vi "Get Element Info Variant.vi"(8 "error in (no error)":errorcluster, 11 "Data Type":variant) -> (0 "error out":errorcluster, 1 "Array Element Size":i32, 2 "Array Size":i32, 3 "Total Size":i32, 4 "Cluster Info":T1[](array[typedef]), 5 "Array":bool)   [LabVIEW 2021, in "CIF_NI_CIPC.lvlib"]
uses:
  CIF_NI_CIPC.lvlib
  <vilib>/CIF Foundation/CIF Utilities/DataTypes/Typedef/Cluster Info.ctl
  <vilib>/Utility/Data Type/Type Definitions/Data Type.ctl
  <vilib>/Utility/Data Type/NI_Data Type.lvlib
  <vilib>/CIF Foundation/CIF Utilities/DataTypes/DataTypes_CIF_U.lvlib
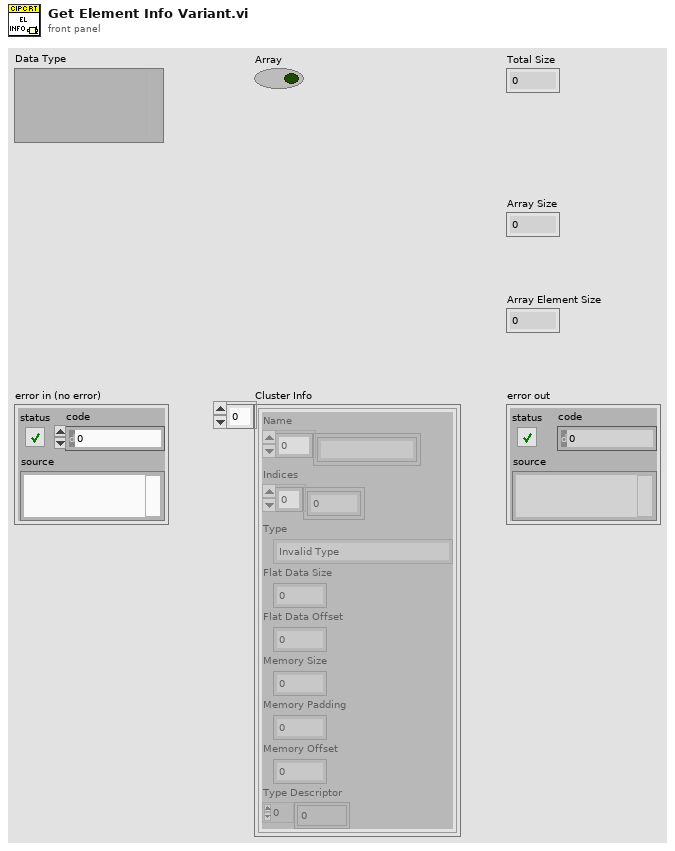
[diagram p1: front panel]
types:
  T1 = typedef "DataTypes_CIF_U.lvlib/Cluster Info.ctl" = cluster{"Name":string[], "Indices":i32[], "Type":T2, "Flat Data Size":u32, "Flat Data Offset":u32, "Memory Size":u32, "Memory Padding":u32, "Memory Offset":u32, "Type Descriptor":i16[]}
  T2 = typedef "NI_Data Type.lvlib/Data Type.ctl" = enum8{"Invalid Type", "Void", "I8", "I16", "I32", "I64", "U8", "U16", "U32", "U64", "Single Float", "Double Float", "Extended Float", "Single Complex", "Double Complex", "Extended Complex", "Enum U8", "Enum U16", "Enum U32", "Enum U64", "Single Float With Unit", "Double Float With Unit", "Extended Float With Unit", "Single Complex with Unit", "Double Complex with Unit", "Extended Complex with Unit", "Boolean", "String", "Path", "Picture", "Tag", "Array", "Cluster", "Variant", "LV Variant", "Waveform", "Timestamp", "Digital Waveform", "Digital Data", "ExpressData", "Refnum", "External Data", "VI", "Poly VI", "LabVIEW Class Instance", "Fixed Point", "Set Collection", "Map Collection"}
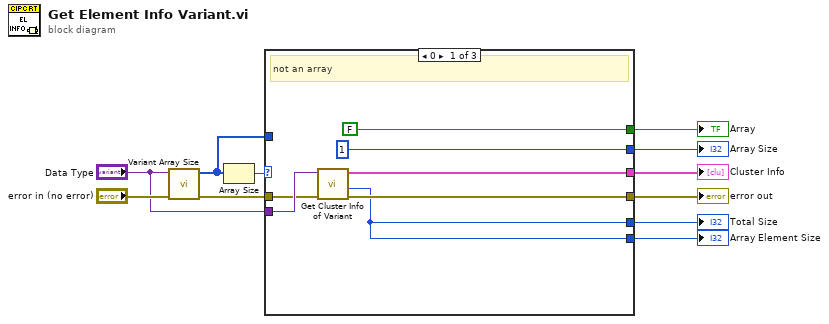
[diagram p0: block diagram]
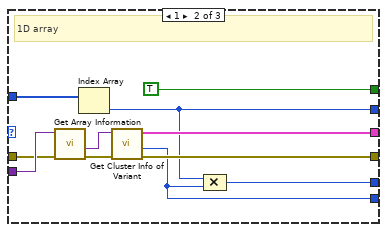
[diagram p2: hidden frame]
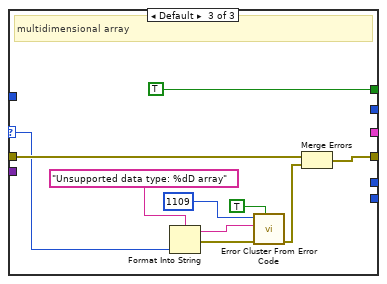
[diagram p3: hidden frame]
diagram:
  n1 = call <vilib>:"Variant Array Size.vi"("error in (no error)"="error in (no error)", "data"="Data Type") -> ("error out"=w9:errorcluster, "lengths"=w1:i32[])  [unwired: 7 in, 1 out]
  n2 = Array Size(array=w1) -> (size(s)=w10:i32)
  n3 = case shown="0" w10 {
    selector: w10 -> [_ _ w31]
    tunnel: w9 -> [w17 w27 w32]
    tunnel: "Data Type" -> [w18 w28 _]
    tunnel: [w16 w24 w30] -> w7
    tunnel: [w12 w21 _] -> w6
    tunnel: [w12 w22 _] -> w5
    tunnel: [w15 w20 _] -> w4
    tunnel: [1 ("array_size") w19 _] -> w3
    tunnel: [FALSE ("is_array?") TRUE ("is_array?") TRUE ("is_array?")] -> w2
    tunnel: w1 -> [_ w23 _]
    frame 0 {
      # "not an array"
      n4 = call <vilib>:"Get Cluster Info of Variant.vi"("error in (no error)"=w17, "Cluster Variant"=w18) -> ("error out"=w16:errorcluster, "mem_size"=w12:i32, "Cluster Info"=w15:T1[])  [unwired: 5 in, 2 out]
    }
    frame 1 {
      # "1D array"
      n5 = call <vilib>:"Get Array Information.vi"("error in (no error)"=w27, "variant"=w28) -> ("error out"=w25:errorcluster, "array element data type"=w26:variant)  [unwired: 6 in, 2 out]
      n6 = Index Array(array=w23) -> (element=w19:i32)  [unwired: 1 in]
      n7 = call <vilib>:"Get Cluster Info of Variant.vi"("error in (no error)"=w25, "Cluster Variant"=w26) -> ("error out"=w24:errorcluster, "mem_size"=w21:i32, "Cluster Info"=w20:T1[])  [unwired: 5 in, 2 out]
      n8 = Compound Arithmetic op=MULTIPLY(w19, w21) -> (w22:i32)
    }
    frame Default {
      # "multidimensional array"
      n9 = Format Into String(format string="Unsupported data type: %dD array", w31) -> (resulting string=w36:string, error out=w34:errorcluster)  [unwired: 2 in]
      n10 = call <vilib>:"Error Cluster From Error Code.vi"("show call chain? (False)"=TRUE, "error in (no error)"=w34, "error message (\"\")"=w36, "error code (0)"=1109) -> ("error out"=w33:errorcluster)  [unwired: 5 in]
      n11 = Merge Errors(w32, w33) -> (w30:errorcluster)
    }
  }
  "Total Size" <- w5
  "Array" <- w2
  "Array Element Size" <- w6
  "error out" <- w7
  "Cluster Info" <- w4
  "Array Size" <- w3
